vi "Cal Step x.vi"(5 "Count":u8, 7 "CalStatus":T1(ring), 9 "Gas Tank":u8, 10 "output cluster 3":T2 {"Current Settings"."Pump" items=["Pump 0", "Pump 1", "Pump 2", "Pump 3", "Pump 4", "Pump 5"]; "Current Settings"."Chart X axis Timescale" min=20 max=180 step=1; "Current Settings"."RunTime Mode Settings"."Exp. Gas Tank" items=["0.07", "0.031", "0.877", "1.863", "3.881", "5.790", "7.688", "6.000"]; "Current Settings"."RunTime Mode Settings"."Insp. Gas Tank" items=["0.07", "0.031", "0.877", "1.863", "3.881", "5.790", "7.688", "6.000"]; "Current Settings"."RunTime Mode Settings"."I:E Ratio" max=30 scale=0.0..7.0; "Current Settings"."RunTime Mode Settings"."Resp Rate Brpm" min=0 max=30 format="%.2f"; "Current Settings"."TE#2 Configuration"."Serial Port"."XOFF Char" format="%.0x"; "Current Settings"."TE#2 Configuration"."Serial Port"."XON Char" format="%.0x"; "Current Settings"."TE#2 Configuration"."Serial Port"."flow control" items=["None"=0, "XON/XOFF"=1, "RTS/CTS"=2, "DTR/DSR"=4]; "Current Settings"."TE#2 Configuration"."Serial Port"."stop bits" items=["1.0"=10, "1.5"=15, "2.0"=20]; "Current Settings"."TE#2 Configuration"."Serial Port"."data bits" min=5 max=8 step=1; "Current Settings"."TE#2 Configuration"."Serial Port"."baud rate" items=["75"=75, "110"=110, "134"=134, "150"=150, "300"=300, "600"=600, "1200"=1200, "1800"=1800, "2400"=2400, "4800"=4800, "7200"=7200, "9600"=9600, "14400"=14400, "19200"=19200, "28800"=28800, "38400"=38400, "56000"=56000, "57600"=57600, "115200"=115200, "128000"=128000, "230400"=230400]; "Current Settings"."TE#2 Configuration"."Serial Port"."termination char" format="%.0x"; "Current Settings"."TE#1 Configuration"."Serial Port"."XOFF Char" format="%.0x"; "Current Settings"."TE#1 Configuration"."Serial Port"."XON Char" format="%.0x"; "Current Settings"."TE#1 Configuration"."Serial Port"."flow control" items=["None"=0, "XON/XOFF"=1, "RTS/CTS"=2, "DTR/DSR"=4]; "Current Settings"."TE#1 Configuration"."Serial Port"."stop bits" items=["1.0"=10, "1.5"=15, "2.0"=20]; "Current Settings"."TE#1 Configuration"."Serial Port"."data bits" min=5 max=8 step=1; "Current Settings"."TE#1 Configuration"."Serial Port"."baud rate" items=["75"=75, "110"=110, "134"=134, "150"=150, "300"=300, "600"=600, "1200"=1200, "1800"=1800, "2400"=2400, "4800"=4800, "7200"=7200, "9600"=9600, "14400"=14400, "19200"=19200, "28800"=28800, "38400"=38400, "56000"=56000, "57600"=57600, "115200"=115200, "128000"=128000, "230400"=230400]; "Current Settings"."TE#1 Configuration"."Serial Port"."termination char" format="%.0x"; "Current Settings"."Capnometer Configuration"."Device" items=["None", "TidalWave", "LoFlow / Canary", "Capnogard"]; "Current Settings"."Capnometer Configuration"."Serial Port"."XOFF Char" format="%.0x"; "Current Settings"."Capnometer Configuration"."Serial Port"."XON Char" format="%.0x"; "Current Settings"."Capnometer Configuration"."Serial Port"."flow control" items=["None"=0, "XON/XOFF"=1, "RTS/CTS"=2, "DTR/DSR"=4]; "Current Settings"."Capnometer Configuration"."Serial Port"."stop bits" items=["1.0"=10, "1.5"=15, "2.0"=20]; "Current Settings"."Capnometer Configuration"."Serial Port"."data bits" min=5 max=8 step=1; "Current Settings"."Capnometer Configuration"."Serial Port"."baud rate" items=["75"=75, "110"=110, "134"=134, "150"=150, "300"=300, "600"=600, "1200"=1200, "1800"=1800, "2400"=2400, "4800"=4800, "7200"=7200, "9600"=9600, "14400"=14400, "19200"=19200, "28800"=28800, "38400"=38400, "56000"=56000, "57600"=57600, "115200"=115200, "128000"=128000, "230400"=230400]; "Current Settings"."Capnometer Configuration"."Serial Port"."termination char" format="%.0x"; "Current Settings"."DAQx Settings"."Analog Output Settings (Volts)" format="%#.3g"; "Current Settings"."DAQx Settings"."Duty Cycle" min=10.0 max=90.0 format="%.1g"; "Current Settings"."DAQx Settings"."Frequency" min=20.0 max=200.0; "Current Settings"."DataLogging Settings"."Data File Duration (Minutes)" min=2 max=200 format="%#.2g"; "Current Settings"."Calibration Settings"."Tolerance #2" min=2 max=4096; "Current Settings"."Calibration Settings"."Cal. Average" min=2 max=4096; "Current Settings"."Test Settings"."Test Sensor ID" items=["(select)", "RB", "YC", "", "Other"]}, 11 "output cluster":T10) -> (2 "New Count":u8, 3 "NewCalStatus":T1(ring))   [LabVIEW 2016]
uses:
  Controls/Cal Refs.ctl
  Controls/DAQ Needed.ctl
  Controls/Processed Variables.ctl
  Controls/AirPump Controls.ctl
  Controls/IE Ratio knob.ctl
  Controls/UI Settings.ctl
  Controls/Aux CO2 Control.ctl
  Controls/Serial Visa Control.ctl
  Controls/Aux CO2 Selector.ctl
  Controls/Aux TE Control.ctl
  Controls/Queues And Others.ctl
  <vilib>/Analysis/baseanly.llb/Mean (DBL).vi
  Miscellaneous/Globals.vi
  <vilib>/Analysis/NI_AALBase.lvlib
panel:
  # "Note: Setting Brpm to zero will\ndisable Insp / Exp digital output."
  # "mmHg"
  # "pts"
  # "tolerance"
  # "AN5 (Temp 1)"
  # "AN6 (Temp 2)"
  # "AN7 (Temp 3)"
  # "AN8 (T FET)"
  # "AN0 (T POT)"
  # "Tref (Set Pt))"
  # "(Spare)"
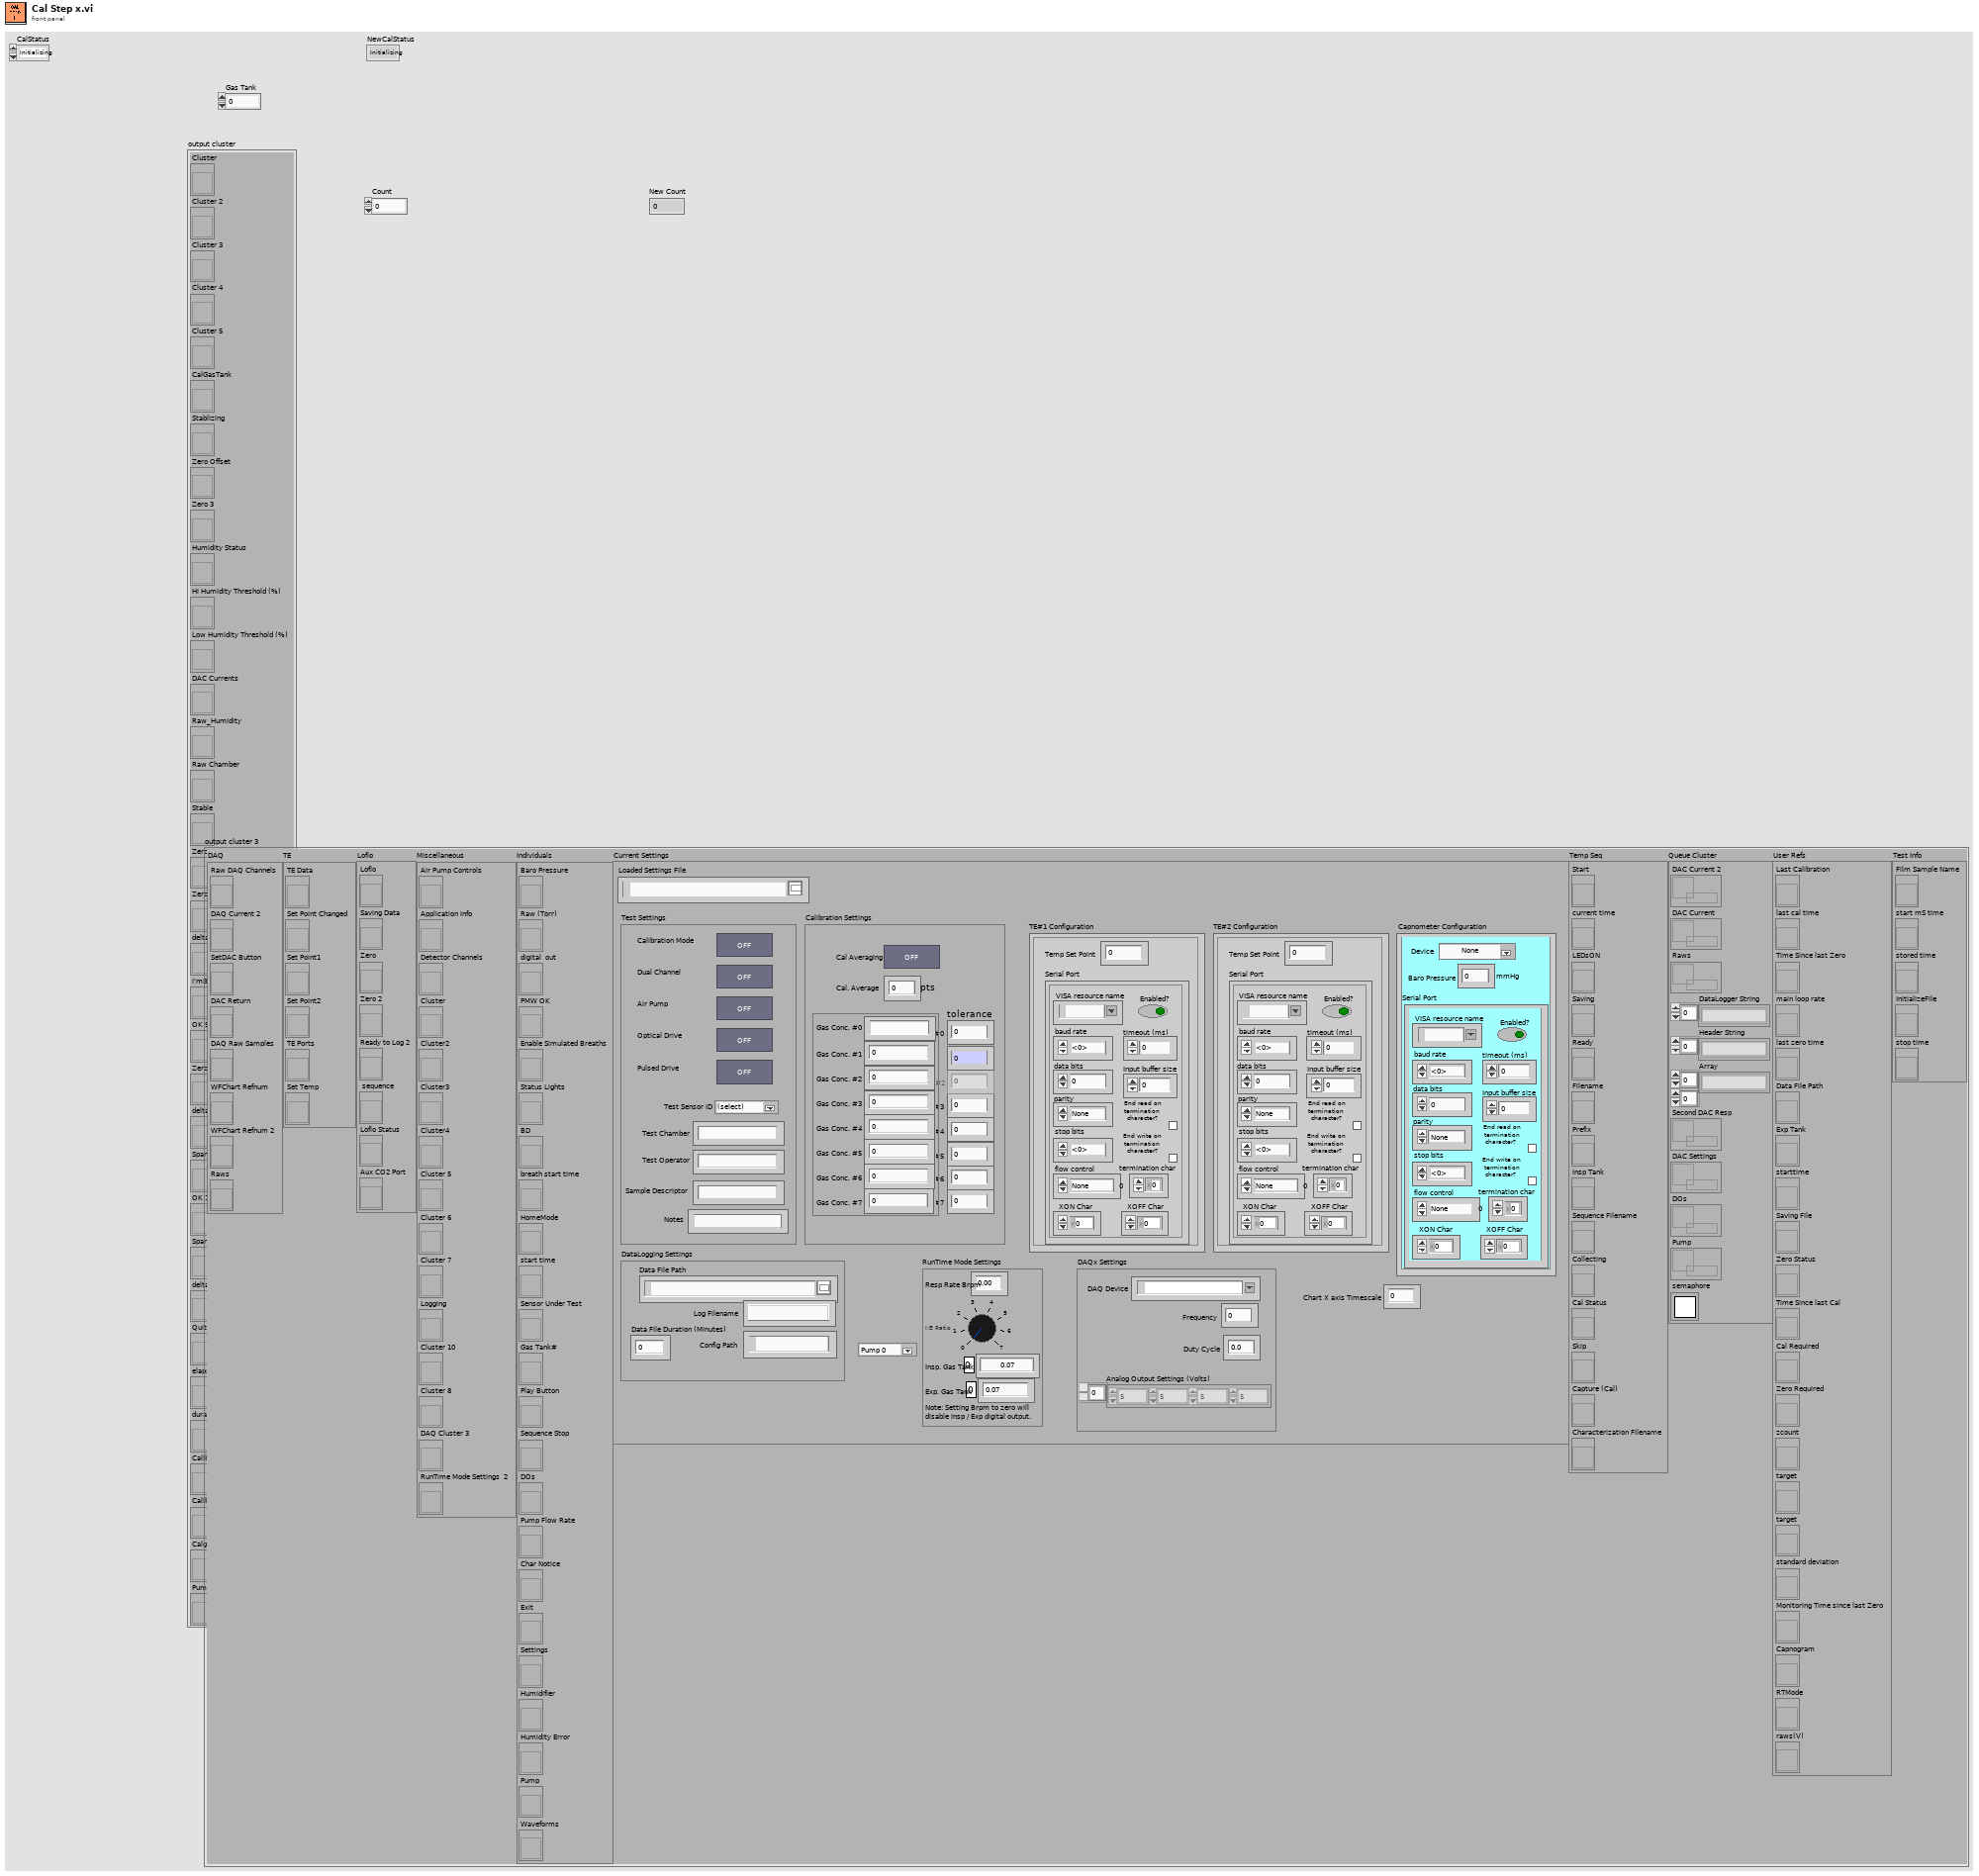
[diagram p1: front panel]
types:
  T1 = enum32{"Initializing", "Enter CO2 Value", "Enter Calibration Code", "Reading Calibration Data", "Stablizing", "Calculating Target Voltages", "Setting Zero Point", "Setting High Point", "Setting Span Point", "Calculating Gain & Offset", "Storing Calibration Coefficients", "Calibration Complete"}
  T2 = typedef "DAQ Needed.ctl" = cluster{"DAQ":cluster{"Raw DAQ Channels":refnum<vi>, "DAQ Current 2":refnum<vi>, "SetDAC Button":refnum<vi>, "DAC Return":refnum<vi>, "DAQ Raw Samples":refnum<vi>, "WFChart Refnum":refnum<vi>, "WFChart Refnum 2":refnum<vi>, "Raws":refnum<vi>}, "TE":cluster{"TE Data":refnum<vi>, "Set Point Changed":refnum<vi>, "Set Point1":refnum<vi>, "Set Point2":refnum<vi>, "TE Ports":refnum<vi>, "Set Temp":refnum<vi>}, "Loflo":cluster{"Loflo":refnum<vi>, "Saving Data":refnum<vi>, "Zero":refnum<vi>, "Zero 2":refnum<vi>, "Ready to Log 2":refnum<vi>, " sequence":refnum<vi>, "Loflo Status ":refnum<vi>, "Aux CO2 Port":refnum<vi>}, "Miscellaneous":cluster{"Air Pump Controls":refnum<vi>, "Application Info":refnum<vi>, "Detector Channels ":refnum<vi>, "Cluster":refnum<vi>, "Cluster2":refnum<vi>, "Cluster3":refnum<vi>, "Cluster4":refnum<vi>, "Cluster 5":refnum<vi>, "Cluster 6":refnum<vi>, "Cluster 7":refnum<vi>, "Logging":refnum<vi>, "Cluster 10":refnum<vi>, "Cluster 8":refnum<vi>, "DAQ Cluster 3":refnum<vi>, "RunTime Mode Settings  2":refnum<vi>}, "Individuals":cluster{"Baro Pressure":refnum<vi>, "Raw (Torr)":refnum<vi>, "digital  out":refnum<vi>, "PMW OK":refnum<vi>, "Enable Simulated Breaths":refnum<vi>, "Status Lights":refnum<vi>, "BD":refnum<vi>, "breath start time":refnum<vi>, "HomeMode":refnum<vi>, "start time":refnum<vi>, "Sensor Under Test":refnum<vi>, "Gas Tank#":refnum<vi>, "Play Button":refnum<vi>, "Sequence Stop":refnum<vi>, "DOs":refnum<vi>, "Pump Flow Rate":refnum<vi>, "Char Notice":refnum<vi>, "Exit":refnum<vi>, "Settings":refnum<vi>, "Humidifier":refnum<vi>, "Humidity Error":refnum<vi>, "Pump":refnum<vi>, "Waveforms":refnum<vi>}, "Current Settings":T3, "Temp Seq":cluster{"Start":refnum<vi>, "current time":refnum<vi>, "LEDsON":refnum<vi>, "Saving":refnum<vi>, "Ready":refnum<vi>, "Filename":refnum<vi>, "Prefix":refnum<vi>, "Insp Tank":refnum<vi>, "Sequence Filename":refnum<vi>, "Collecting":refnum<vi>, "Cal Status":refnum<vi>, "Skip":refnum<vi>, "Capture (Cal)":refnum<vi>, "Characterization Filename":refnum<vi>}, "Queue Cluster":T8, "User Refs":cluster{"Last Calibration":refnum<vi>, "last cal time":refnum<vi>, "Time Since last Zero":refnum<vi>, "main loop rate":refnum<vi>, "last zero time":refnum<vi>, "Data File Path":refnum<vi>, "Exp Tank":refnum<vi>, "starttime":refnum<vi>, "Saving File":refnum<vi>, "Zero Status":refnum<vi>, "Time Since last Cal":refnum<vi>, "Cal Required":refnum<vi>, "Zero Required":refnum<vi>, "zcount":refnum<vi>, "target":refnum<vi>, "target":refnum<vi>, "standard deviation":refnum<vi>, "Monitoring Time since last Zero":refnum<vi>, "Capnogram":refnum<vi>, "RTMode":refnum<vi>, "raws(V)":refnum<vi>}, "Test Info":cluster{"Film Sample Name":refnum<vi>, "start mS time":refnum<vi>, "stored time":refnum<vi>, "InitializeFile":refnum<vi>, "stop time":refnum<vi>}}
  T3 = typedef "UI Settings.ctl" = cluster{"Loaded Settings File":path, "Test Settings":cluster{"Dual Channel":bool, "Air Pump":bool, "Optical Drive":bool, "Pulsed Drive":bool, "Calibration Mode":bool, "Test Sensor ID":u16, "Test Chamber":string, "Test Operator":string, "Sample Descriptor":string, "Notes":string}, "Calibration Settings":cluster{"Cal. Average":u16, "Cal Averaging":bool, "Tolerance #0":sgl, "Tolerance #7":sgl, "Tolerance #6":sgl, "Tolerance #5":sgl, "Tolerance #4":sgl, "Tolerance #3":sgl, "Tolerance #2":sgl, "Tolerance #1":sgl, "Gas Tank Settings":cluster{"Gas Conc. #0":string, "Gas Conc. #1":sgl, "Gas Conc. #2":sgl, "Gas Conc. #3":sgl, "Gas Conc. #4":sgl, "Gas Conc. #5":sgl, "Gas Conc. #6":sgl, "Gas Conc. #7":sgl}}, "DataLogging Settings":cluster{"Data File Path":path, "Data File Duration (Minutes)":sgl, "Log Filename":string, "Config Path":path}, "DAQx Settings":cluster{"DAQ Device":tag, "Frequency":dbl, "Duty Cycle":dbl, "Analog Output Settings (Volts)":sgl[]}, "Capnometer Configuration":T4, "TE#1 Configuration":T7, "TE#2 Configuration":T7, "RunTime Mode Settings ":cluster{"Resp Rate Brpm ":sgl, "I:E Ratio":u8, "Insp. Gas Tank":u16, "Exp. Gas Tank":u16}, "Chart X axis Timescale":u16, "Pump":u16}
  T4 = typedef "Aux CO2 Control.ctl" = cluster{"Serial Port":T5, "Baro Pressure":u32, "Device":T6}
  T5 = typedef "Serial Visa Control.ctl" = cluster{"termination char":u8, "End read on termination character?":bool, "Enabled?":bool, "VISA resource name":refnum<visa-resource-name>, "baud rate":u32, "data bits":u16, "parity":enum16{"None", "Odd", "Even", "Mark", "Space"}, "stop bits":u16, "flow control":u16, "timeout (ms)":u32, "Input buffer size":u32, "End write on termination character?":bool, "XON Char":u8, "XOFF Char":u8}
  T6 = typedef "Aux CO2 Selector.ctl" = u16
  T7 = typedef "Aux TE Control.ctl" = cluster{"Temp Set Point":sgl, "Serial Port":T5}
  T8 = typedef "Queues And Others.ctl" = cluster{"DAC Current 2":refnum<queue>, "DAC Current":refnum<queue>, "Raws":refnum<queue>, "DataLogger String":string[], "Header String":string[], "Array":string[][], "Second DAC Resp":refnum<queue>, "DAC Settings":refnum<queue>, "DOs":refnum<queue>, "Pump":refnum<queue>, "semaphore":T9}
  T9 = typedef "Semaphore RefNum" = refnum<k1>
  T10 = typedef "Cal Refs.ctl" = cluster{"Cluster":refnum<vi>, "Cluster 2":refnum<vi>, "Cluster 3":refnum<vi>, "Cluster 4":refnum<vi>, "Cluster 5":refnum<vi>, "CalGasTank":refnum<vi>, "Stablizing":refnum<vi>, "Zero Offset":refnum<vi>, "Zero 3":refnum<vi>, "Humidity Status":refnum<vi>, "Hi Humidity Threshold (%)":refnum<vi>, "Low Humidity Threshold (%)":refnum<vi>, "DAC Currents":refnum<vi>, "Raw_Humidity":refnum<vi>, "Raw Chamber":refnum<vi>, "Stable":refnum<vi>, "Zero Status":refnum<vi>, "Zero":refnum<vi>, "delta 2":refnum<vi>, "I'mBlue":refnum<vi>, "OK 9":refnum<vi>, "Zero Status 2":refnum<vi>, "delta 3":refnum<vi>, "Span Point Calibration":refnum<vi>, "OK 10":refnum<vi>, "Span Good":refnum<vi>, "delta":refnum<vi>, "Quit":refnum<vi>, "elapsed time":refnum<vi>, "duration":refnum<vi>, "Calibration Complete -":refnum<vi>, "Calibration Complete":refnum<vi>, "Calgas":refnum<vi>, "Pump Settings":refnum<vi>}
  T11 = cluster{"Tcal_Chamber":dbl, "Tcal_PCB":dbl, "Tcal_Film":dbl, "Tcal_Humidity":dbl, "Tcal_Det":dbl[], "Cal Gas":dbl, "Reference":dbl}
  T12 = enum16{"Setting High at 5 mA", "Setting High at 15 mA", "Calculating slopes"}
  T13 = cluster{"CHANNEL 3":string[], "BlueLED 3":bool[], "V_RA(5mA) 2":dbl[], "V_RA(15mA) 2":dbl[], "mI 2":dbl[]}
  T14 = cluster{"CalFile Selected":path, "TYPE":string, "DATE":string, "C0FC2V":dbl[], "C6FC2V":dbl[], "V_0d(target)":dbl[], "V_6d(target)":dbl[], "V_span(target)":dbl[], "CHANNEL":string[], "Status":bool[], "BlueLED 2":bool[], "C2V":u8[], "A":dbl[], "B":dbl[], "C":dbl[], "D":dbl[], "V2C":u8[], "A'":dbl[], "B'":dbl[], "C'":dbl[], "D'":dbl[]}
  T15 = cluster{"CHANNEL 2":string[], "BlueLED":bool[], "V_RA(5mA)":dbl[], "V_RA(15mA)":dbl[], "mI":dbl[], "DAC scale":dbl[]}
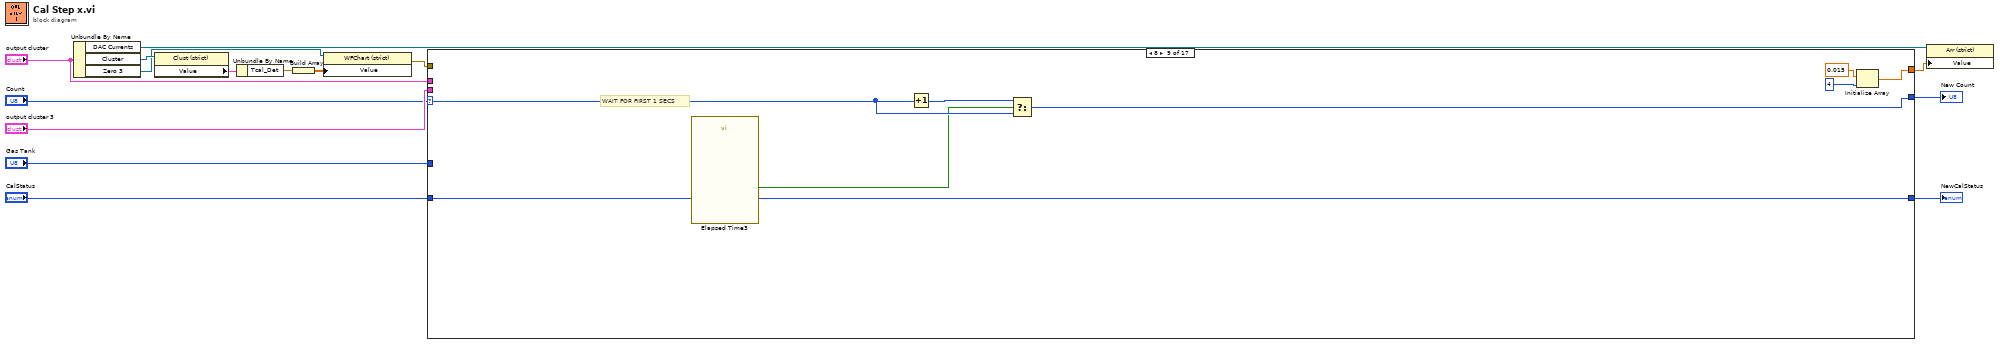
[diagram p0: block diagram]
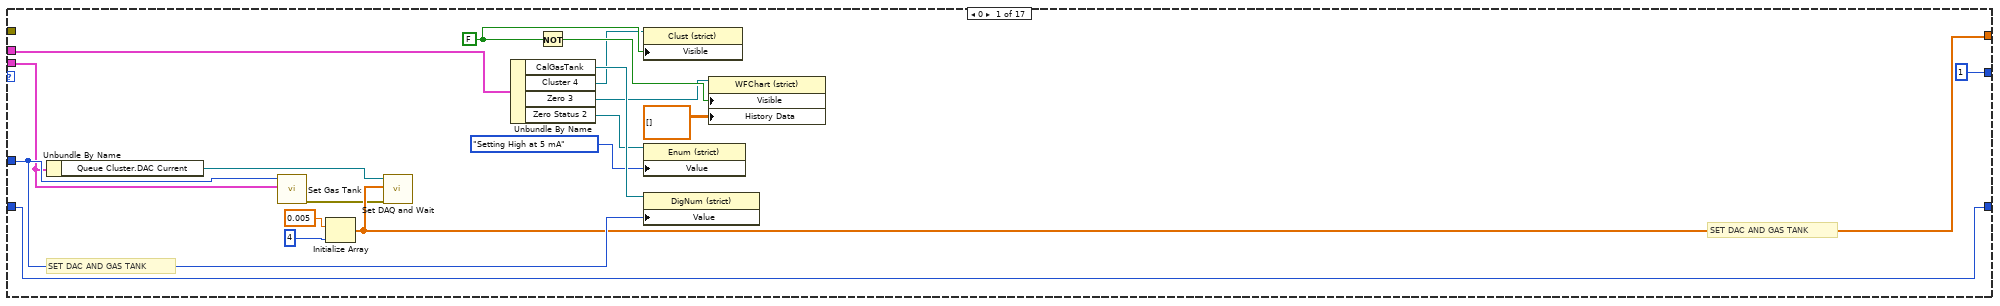
[diagram p2: hidden frame]
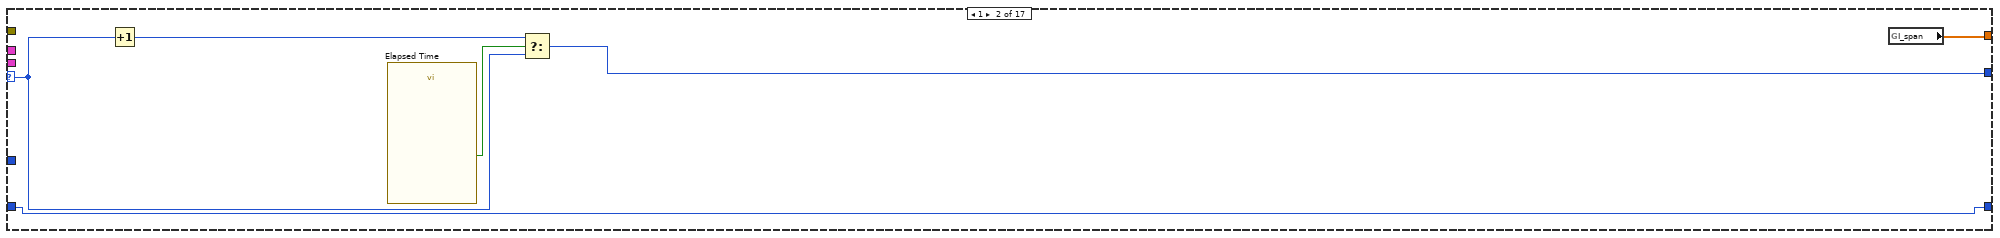
[diagram p3: hidden frame]
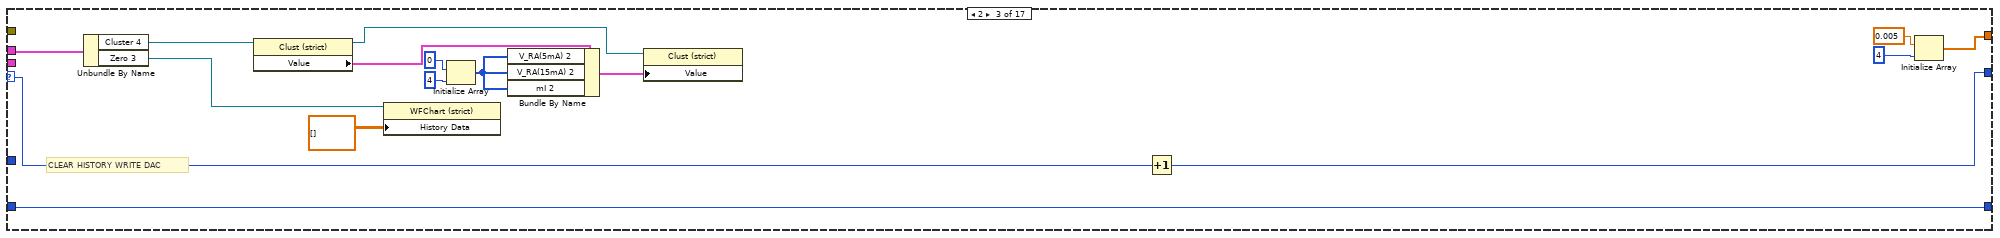
[diagram p4: hidden frame]
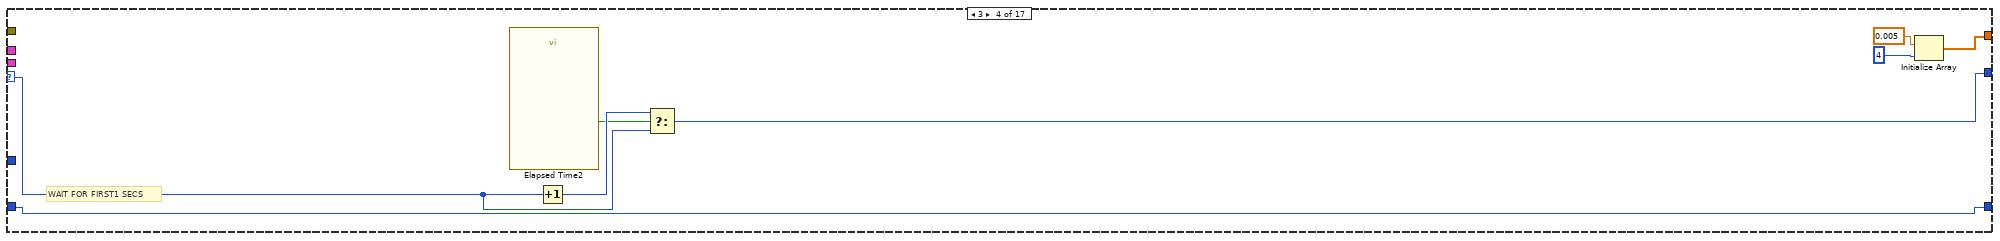
[diagram p5: hidden frame]
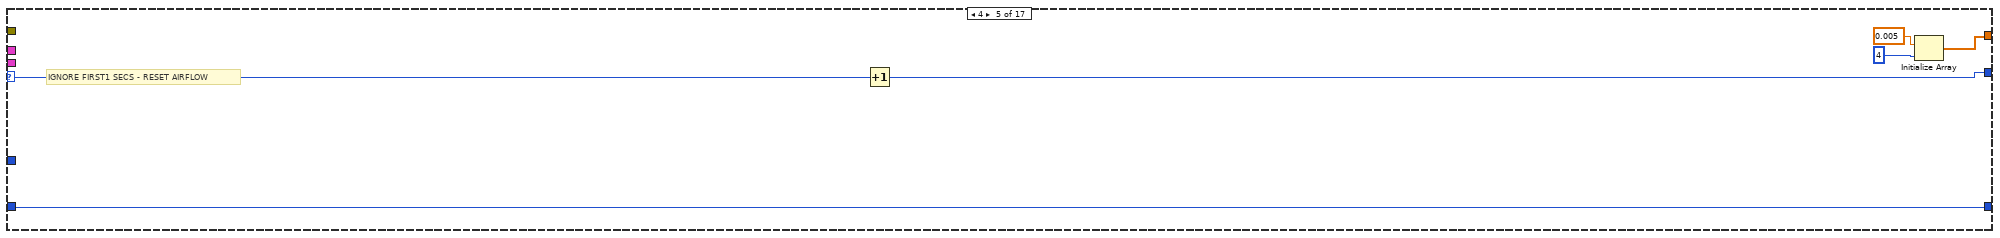
[diagram p6: hidden frame]
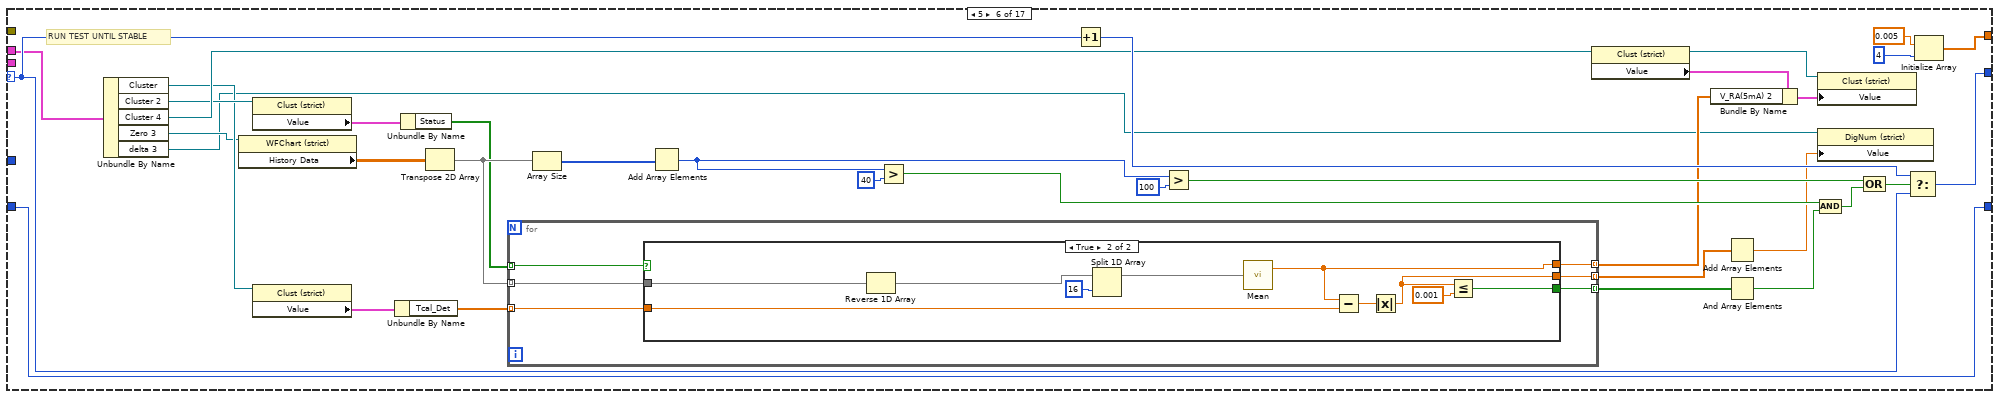
[diagram p7: hidden frame]
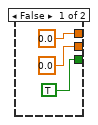
[diagram p8: hidden frame]
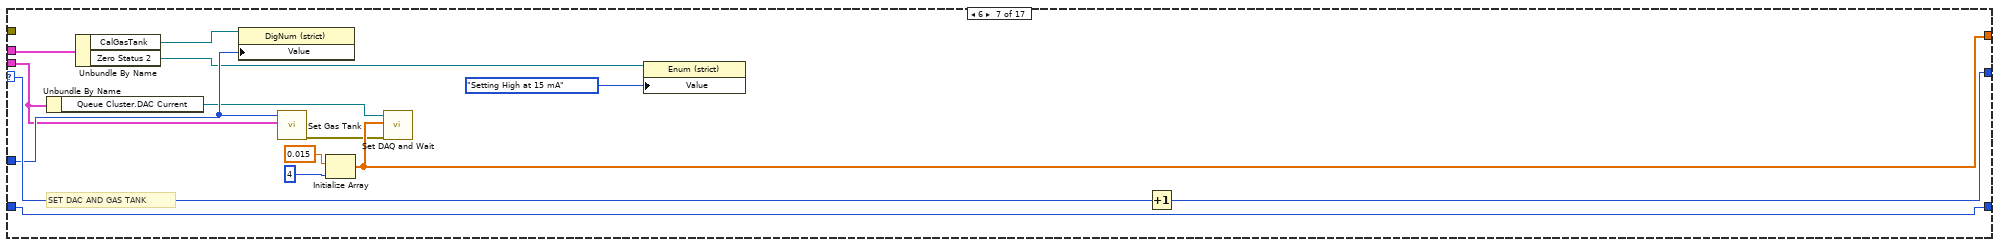
[diagram p9: hidden frame]
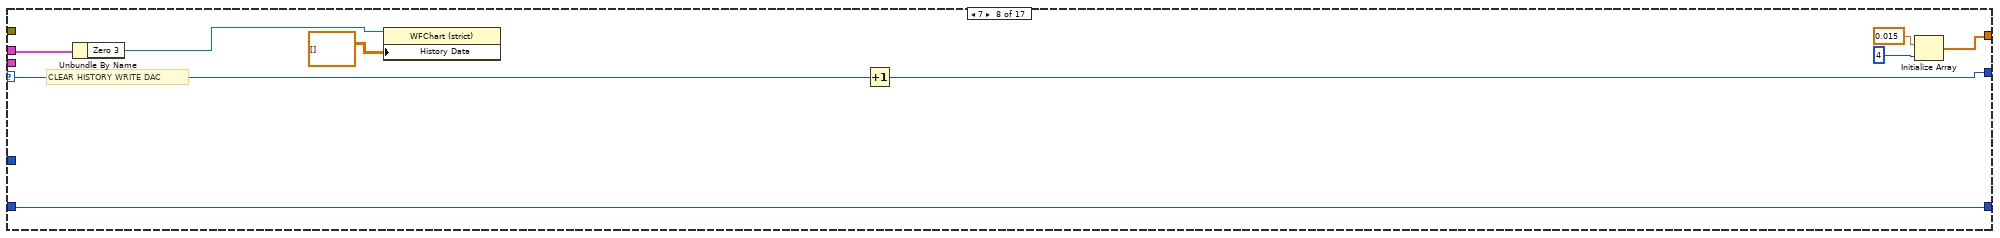
[diagram p10: hidden frame]
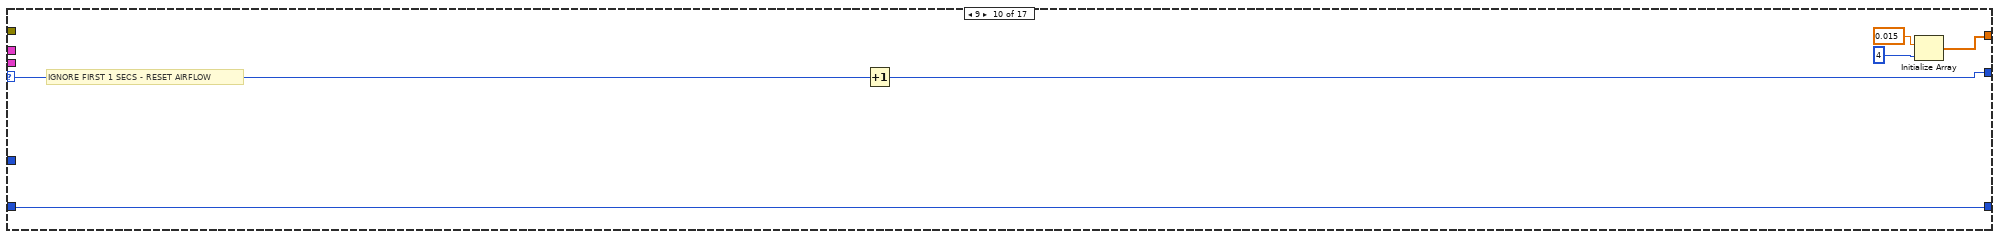
[diagram p11: hidden frame]
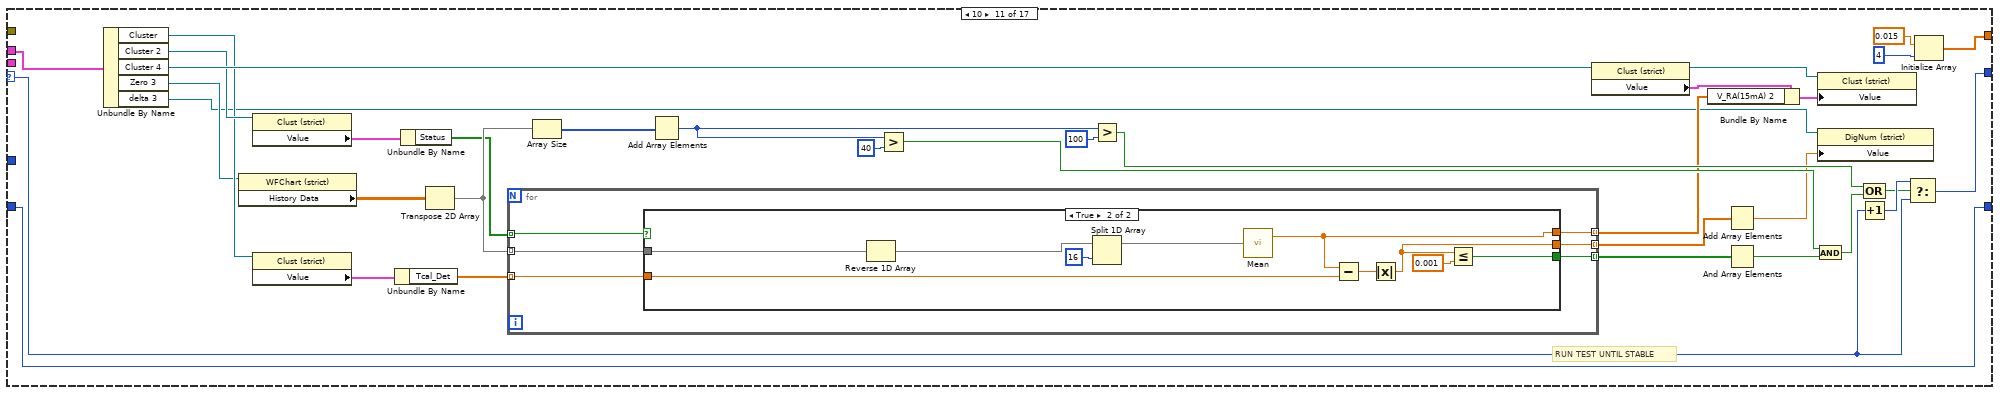
[diagram p12: hidden frame]
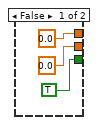
[diagram p13: hidden frame]
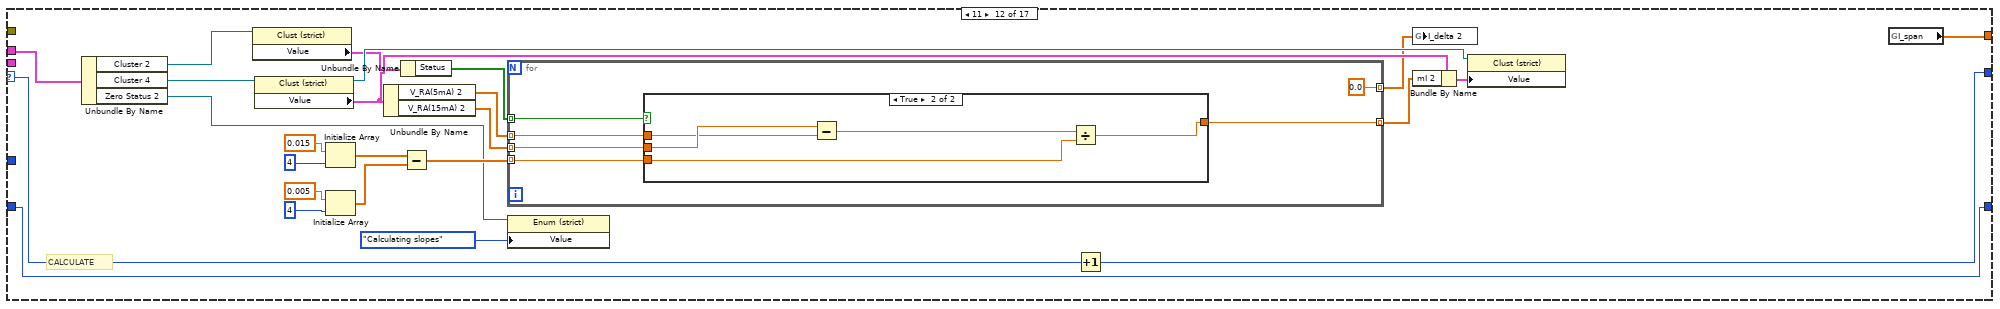
[diagram p14: hidden frame]
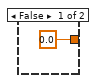
[diagram p15: hidden frame]
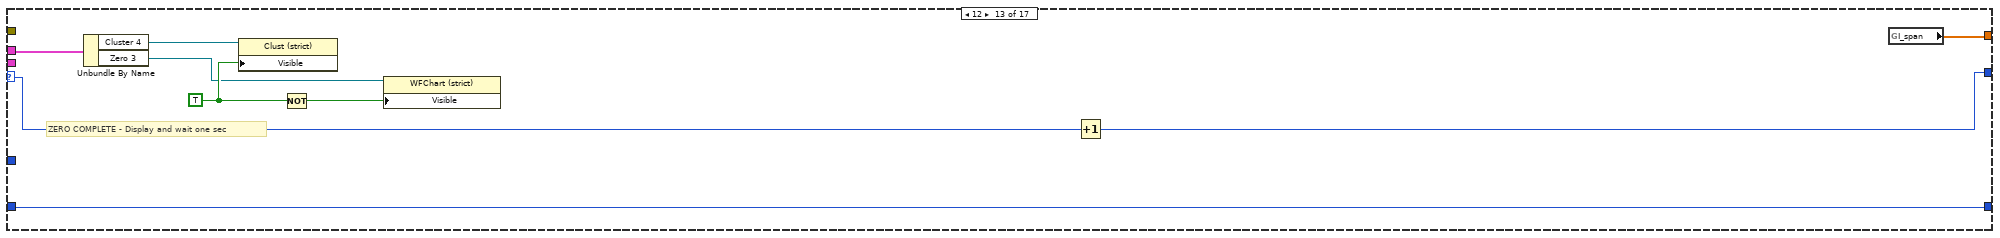
[diagram p16: hidden frame]
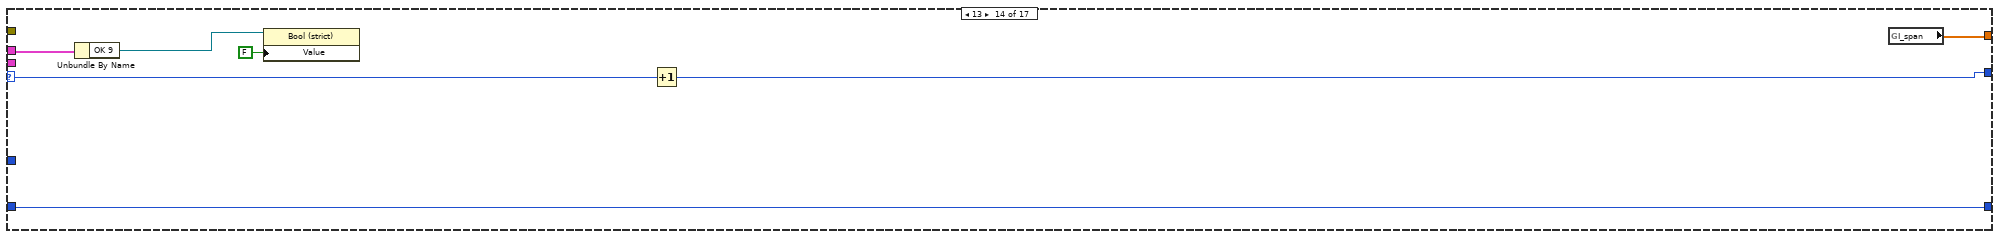
[diagram p17: hidden frame]
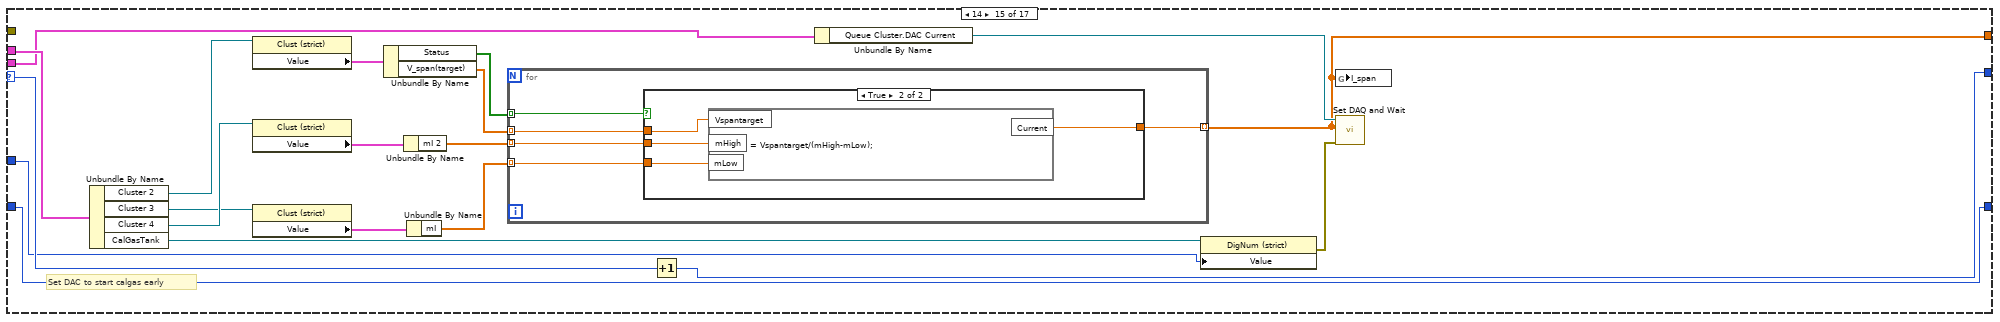
[diagram p18: hidden frame]
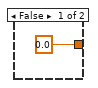
[diagram p19: hidden frame]
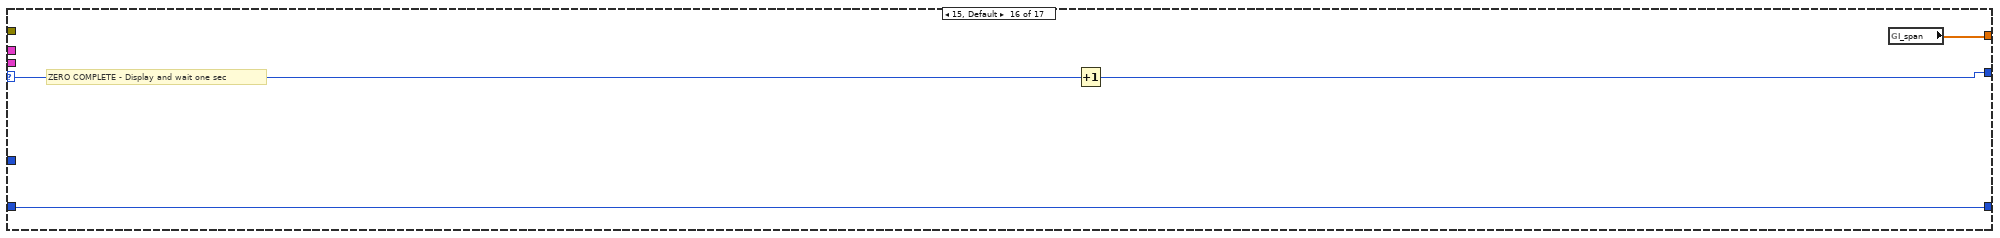
[diagram p20: hidden frame]
diagram:
  n1 = Unbundle By Name("output cluster") -> ("DAC Currents"=w13:refnum<vi>, "Cluster"=w9:refnum<vi>, "Zero 3"=w8:refnum<vi>)
  n2 = property class="Clust (strict)"(reference=w9) -> ("Value"=w11:T11)  [unwired: 1 in, 2 out]
  n3 = Unbundle By Name(w11) -> ("Tcal_Det"=w10:dbl[])
  n4 = Build Array(w10) -> (w7:dbl[][])
  n5 = property class="WFChart (strict)"(reference=w8, "Value"=w7) -> (error out=w6:errorcluster)  [unwired: 1 in, 1 out]
  n6 = case shown="8" "Count" {
    selector: "Count" -> [_ w37 w55 w63 w69 w102 w137 w146 w154 w160 w189 w237 w259 w266 w286 w300 _]
    tunnel: [1 w38 w54 w61 w67 w101 w136 w145 w152 w158 w188 w238 w258 w265 w285 w299 0] -> w1
    tunnel: "CalStatus" -> [w33 w36 w53 w60 w68 w103 w135 w144 w151 w159 w195 w239 w260 w264 w287 w301 w304]
    tunnel: [w33 w36 w53 w60 w68 w103 w135 w144 w151 w159 w195 w239 w260 w264 w287 w301 w303] -> w4
    tunnel: "Gas Tank" -> [w29 _ _ _ _ _ w134 _ _ _ _ _ _ _ w280 _ _]
    tunnel: [w21 w35 w41 w57 w64 w73 w128 w140 w148 w155 w164 w218 w255 w263 w269 w298 w302] -> w12
    tunnel: "output cluster 3" -> [w25 _ _ _ _ _ w130 _ _ _ _ _ _ _ w271 _ _]
    tunnel: "output cluster" -> [w17 _ w45 _ _ w83 w125 w139 _ _ w174 w229 w254 w262 w279 _ _]
    tunnel: w6 -> [_ _ _ _ _ _ _ _ _ _ _ _ _ _ _ _ _]
    frame 0 {
      w30 = FALSE ("Visible")
      # "SET DAC AND GAS TANK"
      # "SET DAC AND GAS TANK"
      n7 = Unbundle By Name(w25) -> ("Queue Cluster.DAC Current"=w20:refnum<queue>)
      n8 = call "Set Gas Tank.vi"("input cluster"=w25, "Gas Tank"=w29) -> ("error out"=w16:errorcluster)  [unwired: 8 in, 1 out]
      n9 = Initialize Array(0.005, 4 ("index")) -> (w21:dbl[])
      n10 = call "Set DAQ and Wait.vi"("error in (no error)"=w16, "Array"=w21, "Queue in"=w20) -> ()  [unwired: 9 in]
      n11 = Unbundle By Name(w17) -> ("CalGasTank"=w28:refnum<vi>, "Cluster 4"=w23:refnum<vi>, "Zero 3"=w19:refnum<vi>, "Zero Status 2"=w18:refnum<vi>)
      n12 = Not(x=w30) -> (.not. x?=w31:bool)
      n13 = property on="Property Node" class="Clust (strict)"(reference=w23, "Visible"=w30) -> ()  [unwired: 1 in, 2 out]
      n14 = property class="Enum (strict)"(reference=w18, "Value"=T12."Setting High at 5 mA" ("Zero Status 2")) -> ()  [unwired: 1 in, 2 out]
      n15 = property class="DigNum (strict)"(reference=w28, "Value"=w29) -> ()  [unwired: 1 in, 2 out]
      n16 = property on="Property Node" class="WFChart (strict)"(reference=w19, "Visible"=w31, "History Data"=dbl[][] []) -> ()  [unwired: 1 in, 2 out]
    }
    frame 1 {
      n17 = Increment(x=w37) -> (x+1=w39:u8)
      n18 = call "Elapsed Time"() -> ("Time has Elapsed"=w34:bool)  [unwired: 12 in, 7 out]
      n19 = Select(t=w39, s=w34, f=w37) -> (s? t:f=w38:u8)
      n20 = global read "Globals.vi" "I_span"() -> (w35:dbl[])
    }
    frame 2 {
      # "CLEAR HISTORY WRITE DAC"
      n21 = Unbundle By Name(w45) -> ("Cluster 4"=w44:refnum<vi>, "Zero 3"=w40:refnum<vi>)
      n22 = property class="Clust (strict)"(reference=w44) -> (reference out=w47:refnum<vi>, "Value"=w48:T13)  [unwired: 1 in, 1 out]
      n23 = property on="Property Node" class="WFChart (strict)"(reference=w40, "History Data"=dbl[][] []) -> ()  [unwired: 1 in, 2 out]
      n24 = Initialize Array(0, 4 ("dimension size")) -> (w46:i32[])
      n25 = Bundle By Name(cluster=w48, "V_RA(5mA) 2"=w46, "V_RA(15mA) 2"=w46, "mI 2"=w46) -> (w49:T13)
      n26 = property class="Clust (strict)"(reference=w47, "Value"=w49) -> ()  [unwired: 1 in, 2 out]
      n27 = Increment(x=w55) -> (x+1=w54:u8)
      n28 = Initialize Array(0.005, 4 ("index")) -> (w41:dbl[])
    }
    frame 3 {
      # "WAIT FOR FIRST1 SECS"
      n29 = call "Elapsed Time2"() -> ("Time has Elapsed"=w56:bool)  [unwired: 12 in, 7 out]
      n30 = Increment(x=w63) -> (x+1=w62:u8)
      n31 = Select(t=w62, s=w56, f=w63) -> (s? t:f=w61:u8)
      n32 = Initialize Array(0.005, 4 ("index")) -> (w57:dbl[])
    }
    frame 4 {
      # "IGNORE FIRST1 SECS - RESET AIRFLOW"
      n33 = Increment(x=w69) -> (x+1=w67:u8)
      n34 = Initialize Array(0.005, 4 ("index")) -> (w64:dbl[])
    }
    frame 5 {
      # "RUN TEST UNTIL STABLE"
      n35 = Unbundle By Name(w83) -> ("Cluster"=w77:refnum<vi>, "Cluster 2"=w81:refnum<vi>, "Cluster 4"=w82:refnum<vi>, "Zero 3"=w71:refnum<vi>, "delta 3"=w70:refnum<vi>)
      n36 = property on="Property Node" class="WFChart (strict)"(reference=w71) -> ("History Data"=w96:dbl[][])  [unwired: 1 in, 2 out]
      n37 = property class="Clust (strict)"(reference=w81) -> ("Value"=w80:T14)  [unwired: 1 in, 2 out]
      n38 = property class="Clust (strict)"(reference=w77) -> ("Value"=w78:T11)  [unwired: 1 in, 2 out]
      n39 = Unbundle By Name(w78) -> ("Tcal_Det"=w76:dbl[])
      n40 = Unbundle By Name(w80) -> ("Status"=w79:bool[])
      n41 = Transpose 2D Array(2D array=w96) -> (transposed array=w95:dbl[][])
      n42 = for {
        tunnel: w95 -> [w110] mode=indexing
        tunnel: w76 -> [w109] mode=indexing
        tunnel: [w108] -> w94 mode=indexing
        tunnel: [w107] -> w84 mode=indexing
        tunnel: [w106] -> w88 mode=indexing
        tunnel: w79 -> [w105] mode=indexing
        n43 = case shown="True" w105 {
          tunnel: w110 -> [_ w118]
          tunnel: w109 -> [_ w117]
          tunnel: [TRUE w116] -> w108
          tunnel: [0.0 ("mean") w115] -> w107
          tunnel: [0.0 w114] -> w106
          frame False {
          }
          frame True {
            n44 = Reverse 1D Array(array=w118) -> (reversed array=w119:dbl[])
            n45 = Split 1D Array(array=w119, index=16) -> (first subarray=w120:dbl[])  [unwired: 1 out]
            n46 = call-poly <vilib>:"Mean.vi"("X"=w120) -> ("mean"=w115:dbl)  [unwired: 1 out]
            n47 = Subtract(x=w115, y=w117) -> (x-y=w122:dbl)
            n48 = Absolute Value(x=w122) -> (abs(x)=w114:dbl)
            n49 = Less Or Equal?(x=w114, y=0.001) -> (x <= y?=w116:bool)
          }
        }
      }
      n50 = Array Size(array=w95) -> (size(s)=w100:i32[])
      n51 = Add Array Elements(numeric array=w100) -> (sum=w89:i32)
      n52 = Greater?(x=w89, y=40 ("index")) -> (0:w98:bool)
      n53 = Increment(x=w102) -> (x+1=w104:u8)
      n54 = Greater?(x=w89, y=100 ("index")) -> (0:w90:bool)
      n55 = property class="Clust (strict)"(reference=w82) -> (reference out=w85:refnum<vi>, "Value"=w86:T13)  [unwired: 1 in, 1 out]
      n56 = Bundle By Name(cluster=w86, "V_RA(5mA) 2"=w84) -> (w87:T13)
      n57 = Add Array Elements(numeric array=w88) -> (sum=w72:dbl)
      n58 = And Array Elements(Boolean array=w94) -> (logical AND=w93:bool)
      n59 = And(x=w98, y=w93) -> (x .and. y?=w91:bool)
      n60 = property class="Clust (strict)"(reference=w85, "Value"=w87) -> ()  [unwired: 1 in, 2 out]
      n61 = property class="DigNum (strict)"(reference=w70, "Value"=w72) -> ()  [unwired: 1 in, 2 out]
      n62 = Compound Arithmetic op=OR(w90, w91) -> (w97:bool)
      n63 = Select(t=w104, s=w97, f=w102) -> (s? t:f=w101:u8)
      n64 = Initialize Array(0.005, 4 ("index")) -> (w73:dbl[])
    }
    frame 6 {
      # "SET DAC AND GAS TANK"
      n65 = Unbundle By Name(w130) -> ("Queue Cluster.DAC Current"=w127:refnum<queue>)
      n66 = Unbundle By Name(w125) -> ("CalGasTank"=w133:refnum<vi>, "Zero Status 2"=w126:refnum<vi>)
      n67 = property class="DigNum (strict)"(reference=w133, "Value"=w134) -> ()  [unwired: 1 in, 2 out]
      n68 = call "Set Gas Tank.vi"("input cluster"=w130, "Gas Tank"=w134) -> ("error out"=w124:errorcluster)  [unwired: 8 in, 1 out]
      n69 = Initialize Array(0.015, 4 ("index")) -> (w128:dbl[])
      n70 = call "Set DAQ and Wait.vi"("error in (no error)"=w124, "Array"=w128, "Queue in"=w127) -> ()  [unwired: 9 in]
      n71 = property class="Enum (strict)"(reference=w126, "Value"=T12."Setting High at 15 mA" ("Zero Status 2")) -> ()  [unwired: 1 in, 2 out]
      n72 = Increment(x=w137) -> (x+1=w136:u8)
    }
    frame 7 {
      # "CLEAR HISTORY WRITE DAC"
      n73 = Unbundle By Name(w139) -> ("Zero 3"=w138:refnum<vi>)
      n74 = property on="Property Node" class="WFChart (strict)"(reference=w138, "History Data"=dbl[][] []) -> ()  [unwired: 1 in, 2 out]
      n75 = Increment(x=w146) -> (x+1=w145:u8)
      n76 = Initialize Array(0.015, 4 ("index")) -> (w140:dbl[])
    }
    frame 8 {
      # "WAIT FOR FIRST 1 SECS"
      n77 = call "Elapsed Time3"() -> ("Time has Elapsed"=w147:bool)  [unwired: 12 in, 7 out]
      n78 = Increment(x=w154) -> (x+1=w153:u8)
      n79 = Select(t=w153, s=w147, f=w154) -> (s? t:f=w152:u8)
      n80 = Initialize Array(0.015, 4 ("index")) -> (w148:dbl[])
    }
    frame 9 {
      # "IGNORE FIRST 1 SECS - RESET AIRFLOW"
      n81 = Increment(x=w160) -> (x+1=w158:u8)
      n82 = Initialize Array(0.015, 4 ("index")) -> (w155:dbl[])
    }
    frame 10 {
      # "RUN TEST UNTIL STABLE"
      n83 = Unbundle By Name(w174) -> ("Cluster"=w168:refnum<vi>, "Cluster 2"=w172:refnum<vi>, "Cluster 4"=w173:refnum<vi>, "Zero 3"=w162:refnum<vi>, "delta 3"=w161:refnum<vi>)
      n84 = property on="Property Node" class="WFChart (strict)"(reference=w162) -> ("History Data"=w187:dbl[][])  [unwired: 1 in, 2 out]
      n85 = property class="Clust (strict)"(reference=w172) -> ("Value"=w171:T14)  [unwired: 1 in, 2 out]
      n86 = property class="Clust (strict)"(reference=w168) -> ("Value"=w169:T11)  [unwired: 1 in, 2 out]
      n87 = Unbundle By Name(w169) -> ("Tcal_Det"=w167:dbl[])
      n88 = Unbundle By Name(w171) -> ("Status"=w170:bool[])
      n89 = Transpose 2D Array(2D array=w187) -> (transposed array=w186:dbl[][])
      n90 = for {
        tunnel: w186 -> [w201] mode=indexing
        tunnel: w167 -> [w200] mode=indexing
        tunnel: [w199] -> w185 mode=indexing
        tunnel: [w198] -> w175 mode=indexing
        tunnel: [w197] -> w179 mode=indexing
        tunnel: w170 -> [w196] mode=indexing
        n91 = case shown="True" w196 {
          tunnel: w201 -> [_ w209]
          tunnel: w200 -> [_ w208]
          tunnel: [TRUE w207] -> w199
          tunnel: [0.0 ("mean") w206] -> w198
          tunnel: [0.0 w205] -> w197
          frame False {
          }
          frame True {
            n92 = Reverse 1D Array(array=w209) -> (reversed array=w210:dbl[])
            n93 = Split 1D Array(array=w210, index=16) -> (first subarray=w211:dbl[])  [unwired: 1 out]
            n94 = call-poly <vilib>:"Mean.vi"("X"=w211) -> ("mean"=w206:dbl)  [unwired: 1 out]
            n95 = Subtract(x=w206, y=w208) -> (x-y=w213:dbl)
            n96 = Absolute Value(x=w213) -> (abs(x)=w205:dbl)
            n97 = Less Or Equal?(x=w205, y=0.001) -> (x <= y?=w207:bool)
          }
        }
      }
      n98 = Array Size(array=w186) -> (size(s)=w193:i32[])
      n99 = Add Array Elements(numeric array=w193) -> (sum=w181:i32)
      n100 = Greater?(x=w181, y=40 ("index")) -> (0:w191:bool)
      n101 = Greater?(x=w181, y=100 ("index")) -> (0:w180:bool)
      n102 = property class="Clust (strict)"(reference=w173) -> (reference out=w176:refnum<vi>, "Value"=w177:T13)  [unwired: 1 in, 1 out]
      n103 = Bundle By Name(cluster=w177, "V_RA(15mA) 2"=w175) -> (w178:T13)
      n104 = Add Array Elements(numeric array=w179) -> (sum=w163:dbl)
      n105 = And Array Elements(Boolean array=w185) -> (logical AND=w184:bool)
      n106 = And(x=w191, y=w184) -> (x .and. y?=w183:bool)
      n107 = property class="Clust (strict)"(reference=w176, "Value"=w178) -> ()  [unwired: 1 in, 2 out]
      n108 = property class="DigNum (strict)"(reference=w161, "Value"=w163) -> ()  [unwired: 1 in, 2 out]
      n109 = Increment(x=w189) -> (x+1=w194:u8)
      n110 = Compound Arithmetic op=OR(w180, w183) -> (w190:bool)
      n111 = Select(t=w194, s=w190, f=w189) -> (s? t:f=w188:u8)
      n112 = Initialize Array(0.015, 4 ("index")) -> (w164:dbl[])
    }
    frame 11 {
      # "CALCULATE"
      n113 = Unbundle By Name(w229) -> ("Cluster 2"=w227:refnum<vi>, "Cluster 4"=w228:refnum<vi>, "Zero Status 2"=w215:refnum<vi>)
      n114 = property class="Clust (strict)"(reference=w227) -> ("Value"=w226:T14)  [unwired: 1 in, 2 out]
      n115 = property class="Clust (strict)"(reference=w228) -> (reference out=w233:refnum<vi>, "Value"=w232:T13)  [unwired: 1 in, 1 out]
      n116 = Initialize Array(0.015, 4 ("index")) -> (w219:dbl[])
      n117 = Initialize Array(0.005, 4 ("index")) -> (w222:dbl[])
      n118 = Unbundle By Name(w232) -> ("V_RA(5mA) 2"=w235:dbl[], "V_RA(15mA) 2"=w234:dbl[])
      n119 = Unbundle By Name(w226) -> ("Status"=w225:bool[])
      n120 = Subtract(x=w219, y=w222) -> (x-y=w236:dbl[])
      n121 = for {
        tunnel: w236 -> [w243] mode=indexing
        tunnel: w235 -> [w244] mode=indexing
        tunnel: w234 -> [w245] mode=indexing
        tunnel: [w242] -> w230 mode=indexing
        tunnel: [0.0 ("x*y")] -> w216 mode=indexing
        tunnel: w225 -> [w240] mode=indexing
        n122 = case shown="True" w240 {
          tunnel: w245 -> [_ w251]
          tunnel: w244 -> [_ w250]
          tunnel: w243 -> [_ w248]
          tunnel: [0.0 w247] -> w242
          frame False {
          }
          frame True {
            n123 = Subtract(x=w251, y=w250) -> (x-y=w249:dbl)
            n124 = Divide(x=w249, y=w248) -> (x/y=w247:dbl)
          }
        }
      }
      n125 = property class="Enum (strict)"(reference=w215, "Value"=T12."Calculating slopes" ("Zero Status 2")) -> ()  [unwired: 1 in, 2 out]
      n126 = Increment(x=w237) -> (x+1=w238:u8)
      n127 = global write "Globals.vi" "I_delta 2"(w216) -> ()
      n128 = Bundle By Name(cluster=w232, "mI 2"=w230) -> (w231:T13)
      n129 = property class="Clust (strict)"(reference=w233, "Value"=w231) -> ()  [unwired: 1 in, 2 out]
      n130 = global read "Globals.vi" "I_span"() -> (w218:dbl[])
    }
    frame 12 {
      w256 = TRUE ("Visible")
      # "ZERO COMPLETE - Display and wait one sec"
      n131 = Unbundle By Name(w254) -> ("Cluster 4"=w253:refnum<vi>, "Zero 3"=w252:refnum<vi>)
      n132 = property on="Property Node" class="Clust (strict)"(reference=w253, "Visible"=w256) -> ()  [unwired: 1 in, 2 out]
      n133 = Not(x=w256) -> (.not. x?=w257:bool)
      n134 = property on="Property Node" class="WFChart (strict)"(reference=w252, "Visible"=w257) -> ()  [unwired: 1 in, 2 out]
      n135 = Increment(x=w259) -> (x+1=w258:u8)
      n136 = global read "Globals.vi" "I_span"() -> (w255:dbl[])
    }
    frame 13 {
      n137 = Unbundle By Name(w262) -> ("OK 9"=w261:refnum<vi>)
      n138 = property class="Bool (strict)"(reference=w261, "Value"=FALSE) -> ()  [unwired: 1 in, 2 out]
      n139 = Increment(x=w266) -> (x+1=w265:u8)
      n140 = global read "Globals.vi" "I_span"() -> (w263:dbl[])
    }
    frame 14 {
      # "Set DAC to start calgas early"
      n141 = Unbundle By Name(w279) -> ("Cluster 2"=w275:refnum<vi>, "Cluster 3"=w276:refnum<vi>, "Cluster 4"=w277:refnum<vi>, "CalGasTank"=w278:refnum<vi>)
      n142 = property class="Clust (strict)"(reference=w275) -> ("Value"=w274:T14)  [unwired: 1 in, 2 out]
      n143 = property class="Clust (strict)"(reference=w277) -> ("Value"=w282:T13)  [unwired: 1 in, 2 out]
      n144 = property class="Clust (strict)"(reference=w276) -> ("Value"=w284:T15)  [unwired: 1 in, 2 out]
      n145 = Unbundle By Name(w274) -> ("Status"=w273:bool[], "V_span(target)"=w272:dbl[])
      n146 = Unbundle By Name(w282) -> ("mI 2"=w281:dbl[])
      n147 = Unbundle By Name(w284) -> ("mI"=w283:dbl[])
      n148 = for {
        tunnel: w283 -> [w292] mode=indexing
        tunnel: [w291] -> w269 mode=indexing
        tunnel: w273 -> [w290] mode=indexing
        tunnel: w281 -> [w289] mode=indexing
        tunnel: w272 -> [w288] mode=indexing
        n149 = case shown="True" w290 {
          tunnel: w292 -> [_ w297]
          tunnel: [0.0 w294] -> w291
          tunnel: w289 -> [_ w296]
          tunnel: w288 -> [_ w295]
          frame False {
          }
          frame True {
            n150 = formula code="Current = Vspantarget/(mHigh-mLow);"("Vspantarget"=w295, "mHigh"=w296, "mLow"=w297) -> ("Current"=w294:dbl)
          }
        }
      }
      n151 = Increment(x=w286) -> (x+1=w285:u8)
      n152 = Unbundle By Name(w271) -> ("Queue Cluster.DAC Current"=w270:refnum<queue>)
      n153 = property class="DigNum (strict)"(reference=w278, "Value"=w280) -> (error out=w268:errorcluster)  [unwired: 1 in, 1 out]
      n154 = global write "Globals.vi" "I_span"(w269) -> ()
      n155 = call "Set DAQ and Wait.vi"("error in (no error)"=w268, "Array"=w269, "Queue in"=w270) -> ()  [unwired: 9 in]
    }
    frame 15, Default {
      # "ZERO COMPLETE - Display and wait one sec"
      n156 = Increment(x=w300) -> (x+1=w299:u8)
      n157 = global read "Globals.vi" "I_span"() -> (w298:dbl[])
    }
    frame 30 {
      n158 = Increment(x=w304) -> (x+1=w303:T1)
      n159 = global read "Globals.vi" "I_span"() -> (w302:dbl[])
    }
  }
  "NewCalStatus" <- w4
  "New Count" <- w1
  n160 = property class="Arr (strict)"(reference=w13, "Value"=w12) -> ()  [unwired: 1 in, 2 out]
